vi "AllianceColorGet.vi"() -> (0 "AllianceColor":T1)   [LabVIEW 2023]
uses:
  <vilib>/Rock Robotics/WPI/DriverStation/WPI_DriverStationAllianceInfo.ctl
  GeneralPurpose/AllianceColorGlobal.vi
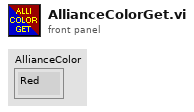
[diagram p1: front panel]
types:
  T1 = typedef "WPI_DriverStationAllianceInfo.ctl" = enum16{"Red", "Blue", "Invalid"}
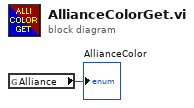
[diagram p0: block diagram]
diagram:
  n1 = global read "AllianceColorGlobal.vi" "Alliance"() -> (→"AllianceColor":T1)
